vi "9dots to parameter.vi"(9 "yDegree":dbl=10.0, 10 "xDegree":dbl=10.0, 11 "9dots":dbl[][](array[numeric])) -> (2 "ScaleArray":T1, 3 "adjutFactor":T2)   [LabVIEW 2011]
uses:
  <vilib>/Analysis/coordinate.llb/2D Cartesian Coordinate Shift (Array).vi
  <vilib>/Analysis/coordinate.llb/2D Cartesian Coordinate Rotation (Array).vi
  <vilib>/Analysis/NI_AALBase.lvlib
  <vilib>/Analysis/NI_AALPro.lvlib
panel:
  out "adjusted":cluster{dbl[], dbl[]}[](graph)
  out "原始图":cluster{dbl[], dbl[]}[](graph)
  out "pupil-CR":dbl[][](array[numeric])
  out "adjutFactor":T3 {"旋转参数" format="%0.2f"}
  out "ScaleArray":dbl[][](array[numeric])
  out "斜率y":dbl[](array[numeric])
  out "旋转后":dbl[][](array[numeric])
  out "slopeY 3":dbl caption="斜率"
  out "slopeY 2":dbl caption="斜率"
  out "slopeY":dbl caption="斜率"
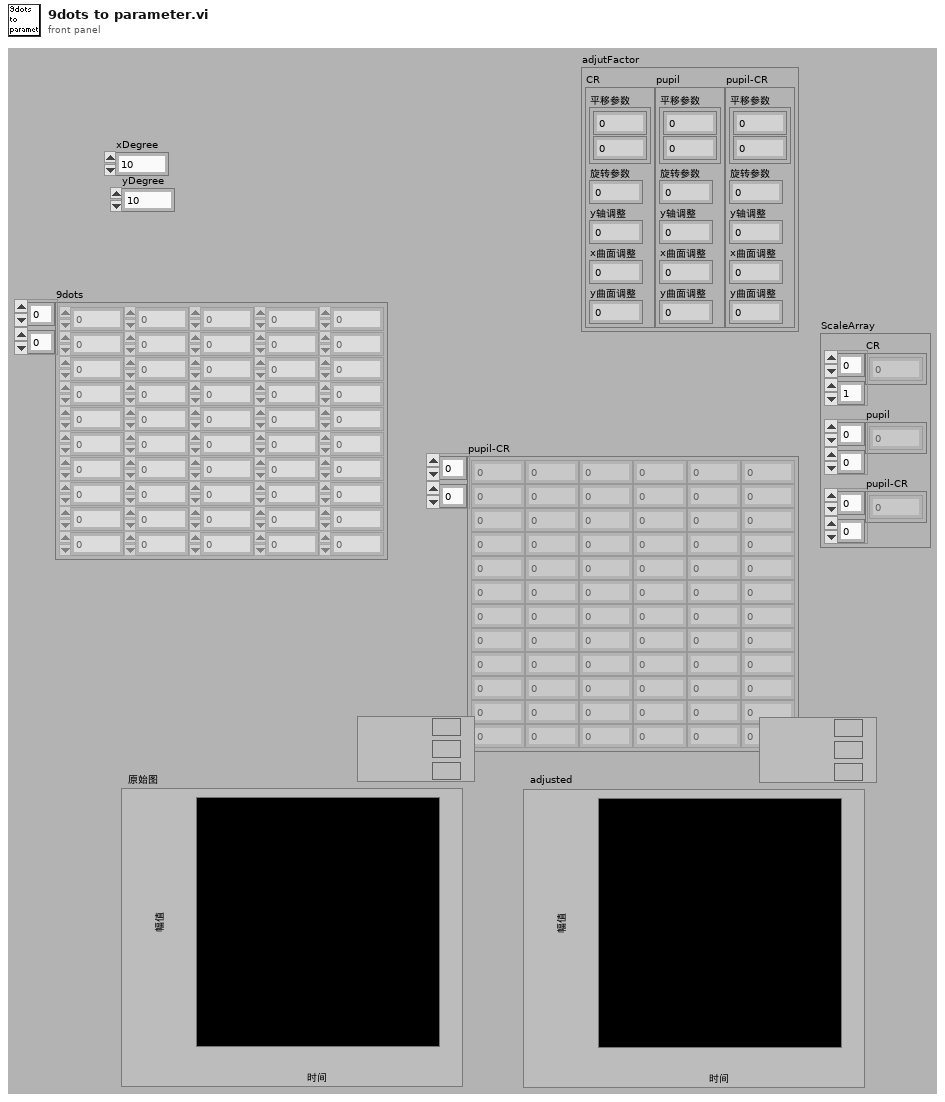
[diagram p1: front panel]
types:
  T1 = cluster{"CR":dbl[][], "pupil":dbl[][], "pupil-CR":dbl[][]}
  T2 = cluster{"CR":cluster{"平移参数":cluster{dbl, dbl}, "旋转参数":dbl, "y轴调整":dbl, "x曲面调整":dbl, "y曲面调整":dbl}, "pupil":cluster{"平移参数":cluster{dbl, dbl}, "旋转参数":dbl, "y轴调整":dbl, "x曲面调整":dbl, "y曲面调整":dbl}, "pupil-CR":cluster{"平移参数":cluster{dbl, dbl}, "旋转参数":dbl, "y轴调整":dbl, "x曲面调整":dbl, "y曲面调整":dbl}}
  T3 = cluster{"平移参数":cluster{dbl, dbl}, "旋转参数":dbl, "y轴调整":dbl, "x曲面调整":dbl, "y曲面调整":dbl}
  T4 = cluster{"adjutFactor":cluster{"平移参数":cluster{dbl, dbl}, "旋转参数":dbl, "y轴调整":dbl, "x曲面调整":dbl, "y曲面调整":dbl}, "adjutFactor":cluster{"平移参数":cluster{dbl, dbl}, "旋转参数":dbl, "y轴调整":dbl, "x曲面调整":dbl, "y曲面调整":dbl}, "adjutFactor":cluster{"平移参数":cluster{dbl, dbl}, "旋转参数":dbl, "y轴调整":dbl, "x曲面调整":dbl, "y曲面调整":dbl}}
  T5 = cluster{"ScaleArray":dbl[][], "ScaleArray":dbl[][], "ScaleArray":dbl[][]}
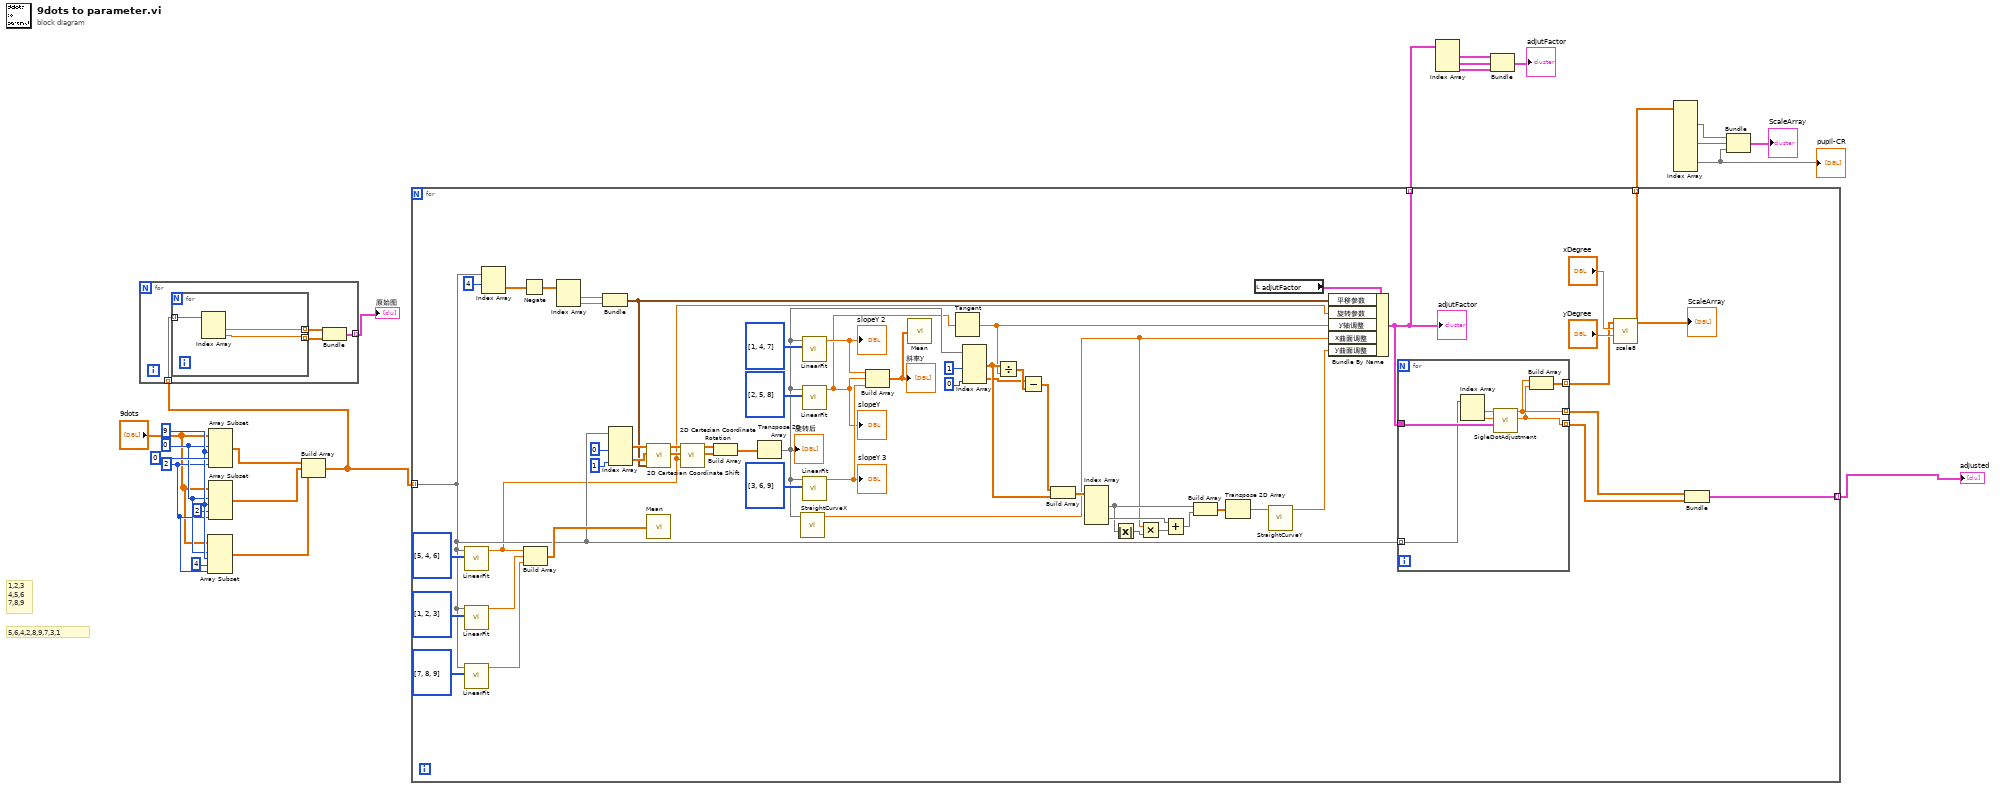
[diagram p0: block diagram]
diagram:
  w13 = 2 ("长度")
  w15 = 9 ("长度")
  w14 = 0 ("索引")
  # "1,2,3\n4,5,6\n7,8,9"
  # "5,6,4,2,8,9,7,3,1"
  n1 = Array Subset(array="9dots", index (row)=w14, length (row)=w15, index (col)=4 ("索引"), length (col)=w13) -> (w2:dbl[][])
  n2 = Array Subset(array="9dots", index (row)=w14, length (row)=w15, index (col)=0 ("索引"), length (col)=w13) -> (w8:dbl[][])
  n3 = Array Subset(array="9dots", index (row)=w14, length (row)=w15, index (col)=2 ("索引"), length (col)=w13) -> (w9:dbl[][])
  n4 = Build Array(w8, w9, w2) -> (w7:dbl[][][])
  n5 = for {
    tunnel: w7 -> [w27] mode=indexing
    tunnel: [w24] -> w6 mode=indexing
    n6 = for {
      tunnel: w27 -> [w30] mode=indexing
      tunnel: [w29] -> w26 mode=indexing
      tunnel: [w28] -> w25 mode=indexing
      n7 = Index Array(array=w30) -> (element #1=w29:dbl, element #2=w28:dbl)  [unwired: 2 in]
    }
    n8 = Bundle(w26, w25) -> (w24:cluster{dbl[], dbl[]})  [unwired: 1 out]
  }
  "原始图" <- w6
  n9 = for {
    tunnel: w7 -> [w39] mode=indexing
    tunnel: [w35] -> w23 mode=indexing
    tunnel: [w34] -> w18 mode=indexing
    tunnel: [w31] -> w5 mode=indexing
    n10 = call "LinearFit.vi"("index"=i32[] [5, 4, 6], "9dots"=w39) -> ("slope"=w37:dbl)  [unwired: 9 out]
    n11 = call "LinearFit.vi"("index"=i32[] [1, 2, 3], "9dots"=w39) -> ("slope"=w42:dbl)  [unwired: 9 out]
    n12 = call "LinearFit.vi"("index"=i32[] [7, 8, 9], "9dots"=w39) -> ("slope"=w41:dbl)  [unwired: 9 out]
    n13 = Index Array(array=w39, index (row)=4 ("索引 (行)")) -> (element=w74:dbl[])  [unwired: 1 in]
    n14 = Negate(x=w74) -> (-x=w73:dbl[])
    n15 = Build Array(w37, w42, w41) -> (w69:dbl[])
    n16 = Index Array(array=w73) -> (element #1=w80:dbl, element #2=w79:dbl)  [unwired: 2 in]
    n17 = Bundle(w80, w79) -> (w52:cluster{dbl, dbl})  [unwired: 1 out]
    n18 = Index Array(array=w39, index (col) #1=0 ("禁用的索引 (列)"), index (col) #2=1 ("索引 (列)")) -> (element #1=w76:dbl[], element #2=w75:dbl[])  [unwired: 2 in]
    n19 = call-poly <vilib>:"2D Cartesian Coordinate Shift.vi"("shift"=w52, "Y"=w75, "X"=w76) -> ("Y Out"=w71:dbl[], "X Out"=w72:dbl[])  [unwired: 7 out]
    n20 = call <vilib>:"Mean.vi"("X"=w69) -> ()  [unwired: 2 out]
    n21 = call-poly <vilib>:"2D Cartesian Coordinate Rotation.vi"("theta"=w37, "Y"=w71, "X"=w72) -> ("Y Out"=w45:dbl[], "X Out"=w46:dbl[])  [unwired: 7 out]
    n22 = Build Array(w46, w45) -> (w70:dbl[][])
    n23 = Transpose 2D Array(2D array=w70) -> (transposed array=w57:dbl[][])
    "旋转后" <- w57
    n24 = call "StraightCurveX.vi"("9dots"=w57) -> ("曲面调整"=w51:dbl)  [unwired: 1 in, 9 out]
    n25 = call "LinearFit.vi"("index"=i32[] [1, 4, 7], "9dots"=w57) -> ("slope"=w44:dbl)  [unwired: 9 out]
    "slopeY 2" <- w44
    n26 = call "LinearFit.vi"("index"=i32[] [2, 5, 8], "9dots"=w57) -> ("slope"=w36:dbl)  [unwired: 9 out]
    "slopeY" <- w36
    n27 = call "LinearFit.vi"("index"=i32[] [3, 6, 9], "9dots"=w57) -> ("slope"=w43:dbl)  [unwired: 9 out]
    "slopeY 3" <- w43
    n28 = Build Array(w44, w36, w43) -> (w55:dbl[])
    "斜率y" <- w55
    n29 = call <vilib>:"Mean.vi"("X"=w55) -> ()  [unwired: 2 out]
    n30 = Tangent(1:w36) -> (0:w40:dbl)
    n31 = Index Array(array=w57, index (col) #1=1 ("禁用的索引 (列)"), index (col) #2=0 ("索引 (列)")) -> (element #1=w48:dbl[], element #2=w47:dbl[])  [unwired: 2 in]
    n32 = Divide(x=w48, y=w40) -> (x/y=w66:dbl[])
    n33 = Subtract(x=w47, y=w66) -> (x-y=w65:dbl[])
    n34 = Build Array(w65, w48) -> (w61:dbl[][])
    n35 = Index Array(array=w61) -> (element #1=w60:dbl[], element #2=w63:dbl[])  [unwired: 4 in]
    n36 = Absolute Value(x=w60) -> (abs(x)=w62:dbl[])
    n37 = Multiply(x=w51, y=w62) -> (x*y=w64:dbl[])
    n38 = Add(x=w63, y=w64) -> (x+y=w59:dbl[])
    n39 = Build Array(w60, w59) -> (w58:dbl[][])
    n40 = Transpose 2D Array(2D array=w58) -> (transposed array=w56:dbl[][])
    n41 = local read "adjutFactor"() -> (w49:T3)
    n42 = call "StraightCurveY.vi"("9dots"=w56) -> ("曲面调整"=w50:dbl)  [unwired: 10 out]
    n43 = Bundle By Name(cluster=w49, "平移参数"=w52, "旋转参数"=w37, "y轴调整"=w40, "x曲面调整"=w51, "y曲面调整"=w50) -> (w35:T3)
    "adjutFactor" <- w35
    n44 = for {
      tunnel: w35 -> [w94]
      tunnel: w39 -> [w93] mode=indexing
      tunnel: [w90] -> w38 mode=indexing
      tunnel: [w89] -> w33 mode=indexing
      tunnel: [w88] -> w32 mode=indexing
      n45 = Index Array(array=w93) -> (element #1=w92:dbl, element #2=w91:dbl)  [unwired: 2 in]
      n46 = call "SigleDotAdjustment.vi"("adjutFactor"=w94, "y"=w91, "x"=w92) -> ("y"=w88:dbl, "x"=w89:dbl)  [unwired: 7 out]
      n47 = Build Array(w89, w88) -> (w90:dbl[])
    }
    n48 = call "scale8.vi"("yDegree"="yDegree", "xDegree"="xDegree", "9dots"=w38) -> ("ScaleArray"=w34:dbl[][])  [unwired: 8 out]
    "ScaleArray" <- w34
    n49 = Bundle(w33, w32) -> (w31:cluster{dbl[], dbl[]})  [unwired: 1 out]
  }
  "adjusted" <- w5
  n50 = Index Array(array=w23) -> (element #1=w22:T3, element #2=w21:T3, element #3=w20:T3)  [unwired: 3 in]
  n51 = Bundle("adjutFactor"=w22, "adjutFactor"=w21, "adjutFactor"=w20) -> (→"adjutFactor":T4)  [unwired: 1 out]
  n52 = Index Array(array=w18) -> (element #1=w3:dbl[][], element #2=w4:dbl[][], element #3=w1:dbl[][])  [unwired: 9 in]
  "pupil-CR" <- w1
  n53 = Bundle("ScaleArray"=w3, "ScaleArray"=w4, "ScaleArray"=w1) -> (→"ScaleArray":T5)  [unwired: 1 out]
